vi "Main.vi"() -> ()   [LabVIEW 2018]
uses:
  <vilib>/picture/picture.llb/imagedata.ctl
panel:
  out "out":picture
  out "size(s)":i32[](array[numeric])
  out "24-bit pixmap":u32[][](array[numeric]) format="%x"
  out "new picture":picture
  in  "path to PNG file":path=path "D:/LabVIEW Work/Pets/Waterfall/pops.png"
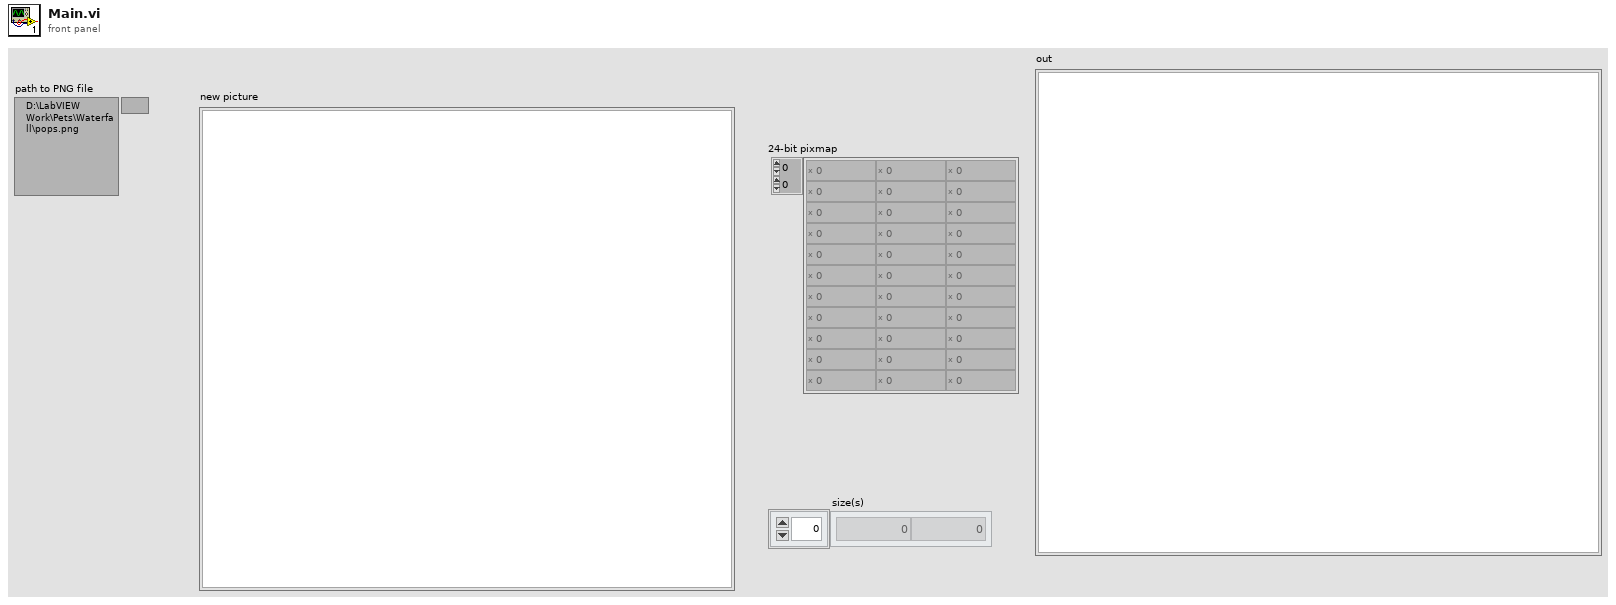
[diagram p1: front panel]
types:
  T1 = typedef "imagedata.ctl" = cluster{"image type":i32, "image depth":i32, "image":u8[], "mask":u8[], "colors":u32[], "Rectangle":cluster{"left":i16, "top":i16, "right":i16, "bottom":i16}}
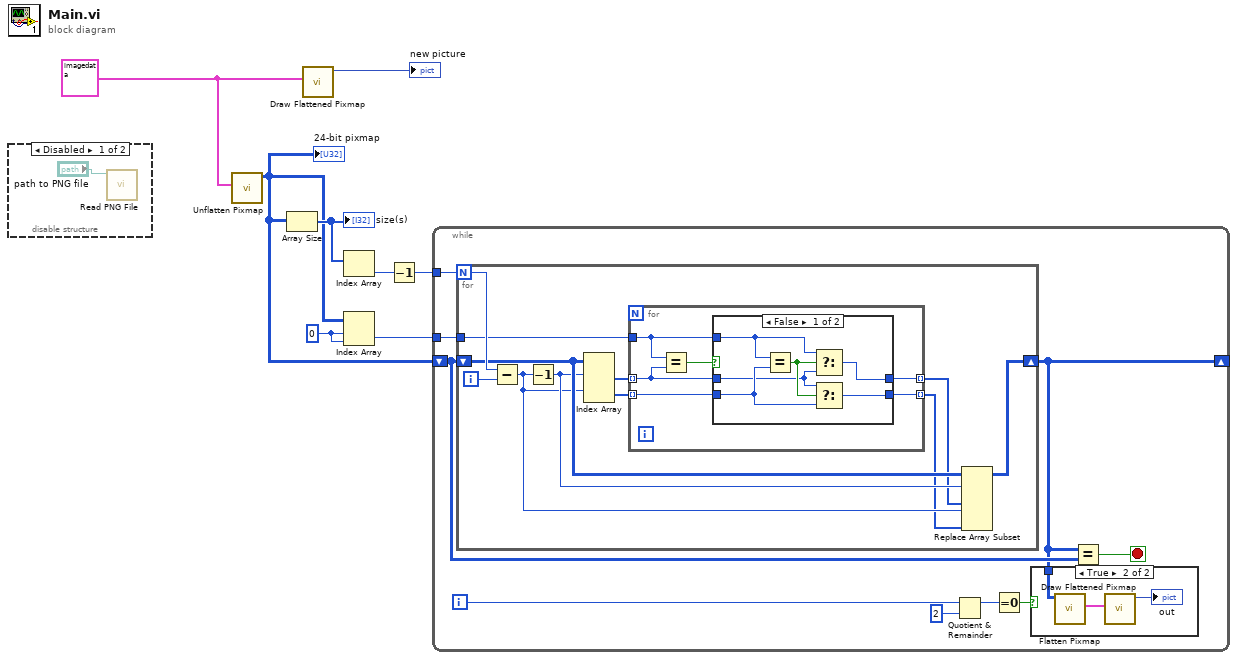
[diagram p0: block diagram]
diagram:
  w1 = T1 {"image type"=0, "image depth"=24, "image"=array[740862 elements], "mask"=[], "colors"=[], "Rectangle"={"left"=0, "top"=0, "right"=521, "bottom"=474}} ("image data")
  w7 = 0 ("index (row)")
  n1 = disable-structure shown="Disabled" {
    frame Disabled {
      n2 = call <vilib>:"Read PNG File.vi"("path to PNG file"="path to PNG file") -> ()  [unwired: 8 in, 3 out]
    }
    frame Enabled {
    }
  }
  n3 = call <vilib>:"Unflatten Pixmap.vi"("image data"=w1) -> ("24-bit pixmap"=w5:u32[][])  [unwired: 4 in, 6 out]
  "24-bit pixmap" <- w5
  n4 = Array Size(array=w5) -> (size(s)=w6:i32[])
  "size(s)" <- w6
  n5 = call <vilib>:"Draw Flattened Pixmap.vi"("image data"=w1) -> ("new picture"=→"new picture":picture)  [unwired: 8 in]
  n6 = Index Array(array=w6) -> (element=w4:i32)  [unwired: 1 in]
  n7 = Index Array(array=w5, index (row)=w7, index (col)=w7) -> (element=w2:u32)
  n8 = Decrement(x=w4) -> (x-1=w3:i32)
  n9 = while {
    tunnel: w3 -> [w18]
    tunnel: w2 -> [w17]
    shift-right: [w14] -> _
    shift-left: w5 -> [w16]
    i -> [w13]
    stop <- w15 stop-if-true
    n10 = for {
      N: w18 -> [w32]
      tunnel: w17 -> [w28]
      shift-right: [w22] -> w14
      shift-left: w16 -> [w27]
      i -> [w31]
      n11 = Subtract(x=w32, y=w31) -> (x-y=w24:i32)
      n12 = Decrement(x=w24) -> (x-1=w26:i32)
      n13 = Index Array(array=w27, index (row) #1=w26, index (row) #2=w24) -> (element #1=w30:u32[], element #2=w29:u32[])  [unwired: 2 in]
      n14 = for {
        tunnel: w30 -> [w36] mode=indexing
        tunnel: w28 -> [w33]
        tunnel: w29 -> [w37] mode=indexing
        tunnel: [w35] -> w25 mode=indexing
        tunnel: [w34] -> w23 mode=indexing
        n15 = Equal?(x=w33, y=w36) -> (x = y?=w38:bool)
        n16 = case shown="False" w38 {
          tunnel: w37 -> [w44 w45]
          tunnel: w36 -> [w39 w46]
          tunnel: [w42 w46] -> w35
          tunnel: [w43 w45] -> w34
          tunnel: w33 -> [w40 _]
          frame False {
            n17 = Equal?(x=w40, y=w44) -> (x = y?=w41:bool)
            n18 = Select(t=w40, s=w41, f=w39) -> (s? t:f=w42:u32)
            n19 = Select(t=w39, s=w41, f=w44) -> (s? t:f=w43:u32)
          }
          frame True {
          }
        }
      }
      n20 = Replace Array Subset(array=w27, new element #1=w25, index (row) #1=w26, new element #2=w23, index (row) #2=w24) -> (w22:u32[][])  [unwired: 2 in]
    }
    n21 = Quotient & Remainder(x=w13, y=2) -> (x-y*floor(x/y)=w10:i32)  [unwired: 1 out]
    n22 = Equal To 0?(x=w10) -> (x = 0?=w11:bool)
    n23 = case shown="True" w11 {
      tunnel: w14 -> [_ w19]
      frame False {
      }
      frame True {
        n24 = call <vilib>:"Flatten Pixmap.vi"("24-bit pixmap"=w19) -> ("image data"=w21:T1)  [unwired: 10 in]
        n25 = call <vilib>:"Draw Flattened Pixmap.vi"("image data"=w21) -> ("new picture"=→"out":picture)  [unwired: 8 in]
      }
    }
    n26 = Equal?(x=w14, y=w16) -> (x = y?=w15:bool)
  }
